vi "Cam W.vi"() -> ()   [LabVIEW 2016]
panel:
  out "Cam W":dbl
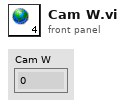
[diagram p1: front panel]
diagram:
